vi "RT Loop - Data Logging.vi"(0 "Message Queues":T1 caption="消息队列", 3 "error in (no error)":errorcluster caption="错误输入（无错误）") -> (10 "error out":errorcluster caption="错误输出")   [LabVIEW 2015]
uses:
  Support VIs/Message Queue/All Real-Time Message Queues.ctl
  Support VIs/Message Queue/Message Cluster.ctl
  Globals/Global - All RT Loop Stop.vi
  Globals/Global - Monitoring Variables.vi
  Globals/Global - RT Stream Connections.vi
  Globals/Global - Configuration Options.vi
  Support VIs/Message Queue/Message Queue.lvlib
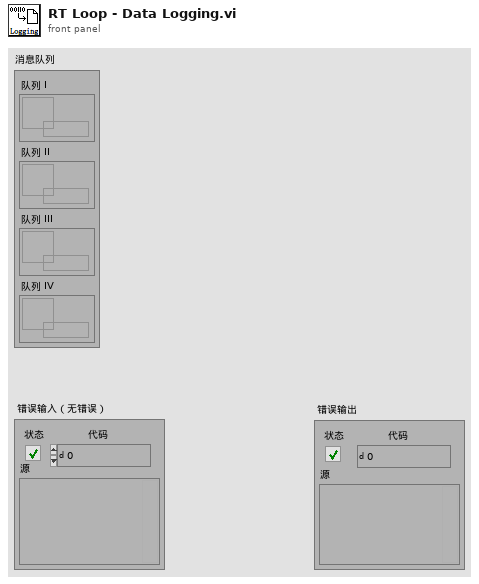
[diagram p1: front panel]
types:
  T1 = typedef "Message Queue.lvlib/All Real-Time Message Queues.ctl" = cluster{"Queue I":refnum<queue>, "Queue II":refnum<queue>, "Queue III":refnum<queue>, "Queue IV":refnum<queue>}
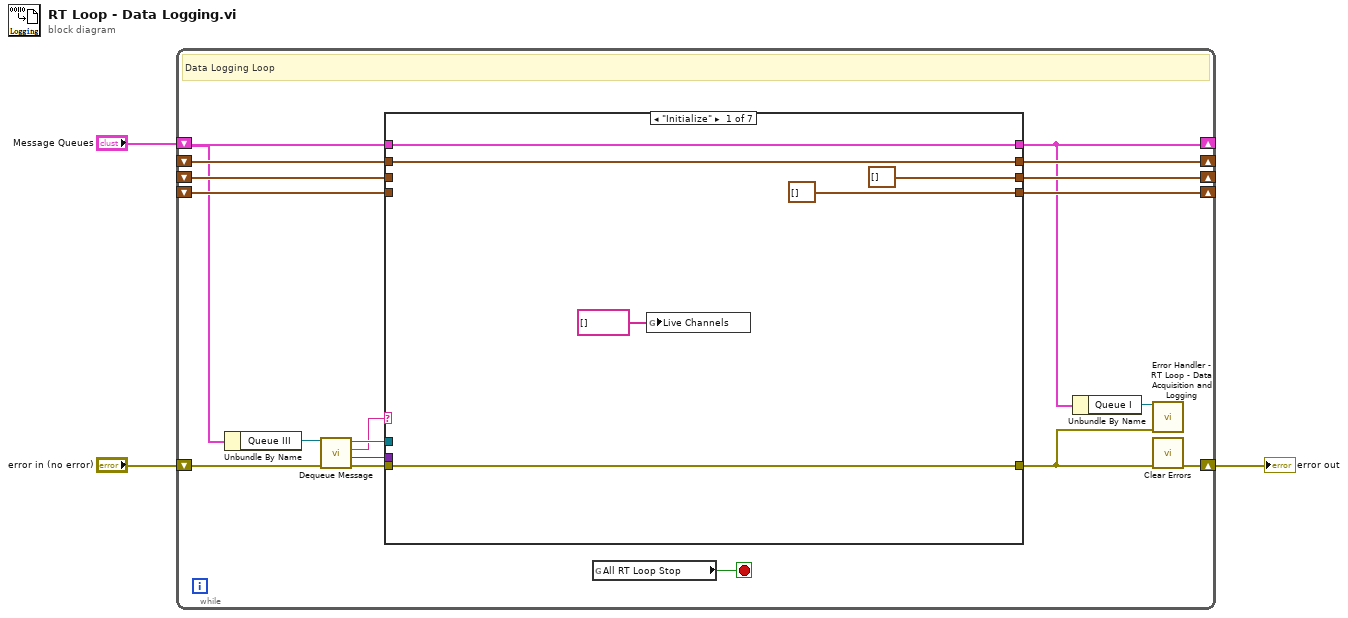
[diagram p0: block diagram]
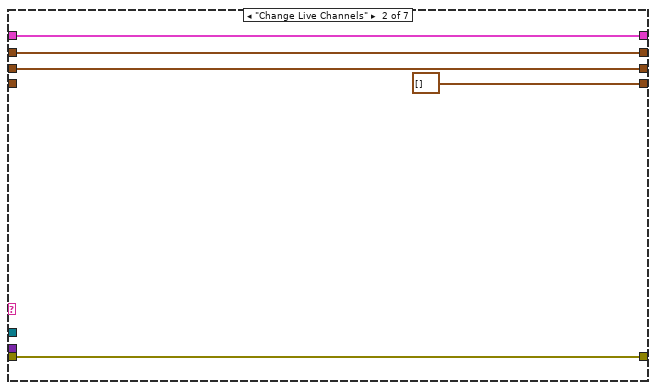
[diagram p2: hidden frame]
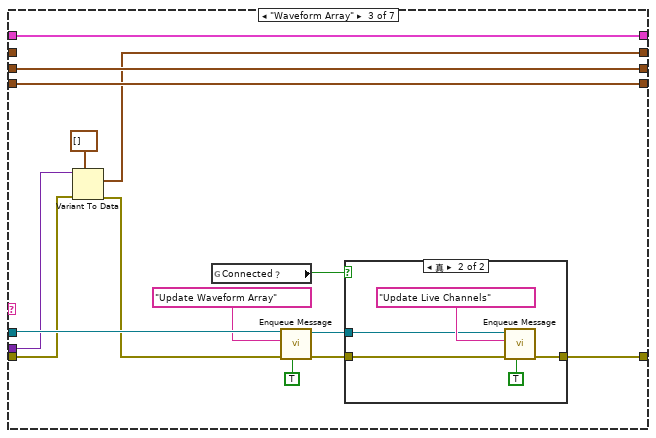
[diagram p3: hidden frame]
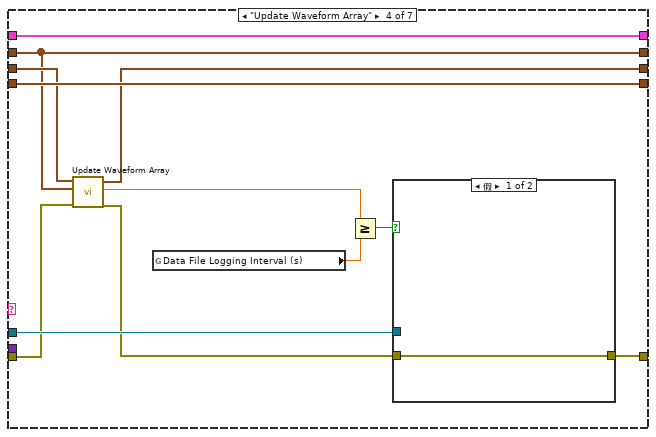
[diagram p5: hidden frame]
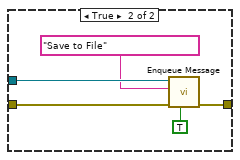
[diagram p6: hidden frame]
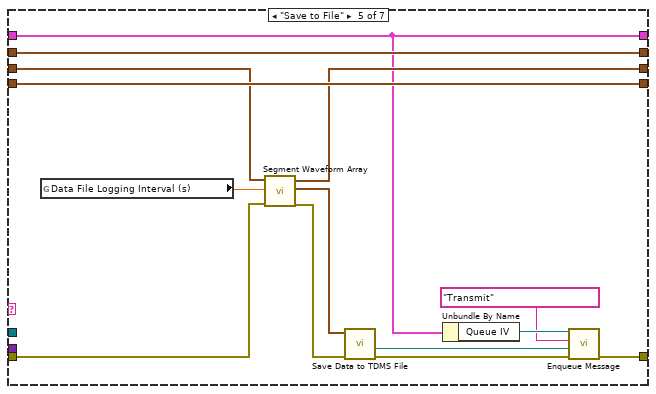
[diagram p7: hidden frame]
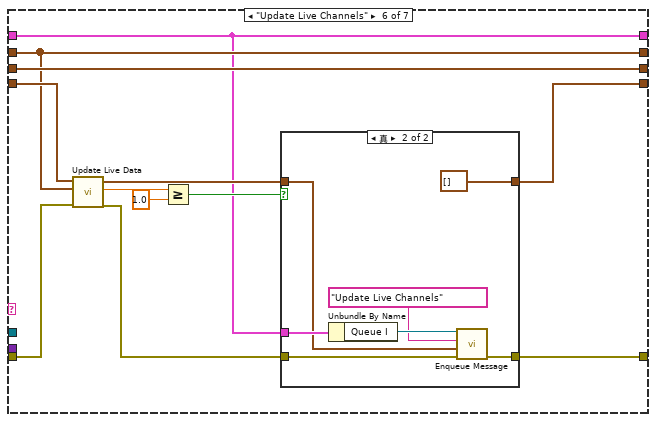
[diagram p8: hidden frame]
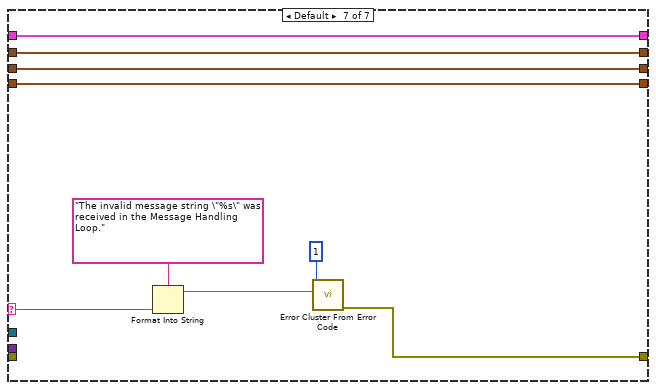
[diagram p10: hidden frame]
diagram:
  n1 = while {
    shift-right: [w17] -> _
    shift-left: _ -> [w10]
    shift-right: [w6] -> _
    shift-left: "Message Queues" -> [w7]
    shift-right: [w16] -> _
    shift-left: _ -> [w11]
    shift-right: [w12] -> w3
    shift-left: "error in (no error)" -> [w18]
    shift-right: [w8] -> _
    shift-left: _ -> [w9]
    stop <- w21 stop-if-true
    # "Data Logging Loop"
    n2 = Unbundle By Name(w7) -> ("Queue III"=w15:refnum<queue>)
    n3 = call "Dequeue Message.vi"("error in (no error)"=w18, "Message Queue"=w15) -> ("error out"=w20:errorcluster, "Message Data"=w19:variant, "Message"=w4:string, "dup Message Queue"=w5:refnum<queue>)  [unwired: 6 in]
    n4 = case shown="\"Initialize\"" w4 {
      tunnel: w19 -> [_ _ w45 _ _ _ _]
      selector: w4 -> [_ _ _ _ _ _ w112]
      tunnel: w20 -> [w24 w29 w46 w63 w77 w96 _]
      tunnel: [w26 w31 w33 w55 w80 w90 w109] -> w17
      tunnel: [w24 w29 w39 w58 w83 w97 w111] -> w13
      tunnel: w10 -> [w26 w31 _ w55 w80 w90 w109]
      tunnel: w7 -> [w27 w32 w35 w54 w72 w87 w110]
      tunnel: [w27 w32 w35 w54 w72 w87 w110] -> w6
      tunnel: [waveform(dbl)[] [] waveform(dbl)[] [] w43 w64 w85 w86 w108] -> w16
      tunnel: w11 -> [_ _ w43 w64 w85 w94 w108]
      tunnel: w9 -> [_ w30 w34 w62 w79 w91 w107]
      tunnel: [waveform(dbl)[] [] w30 w34 w61 w76 w91 w107] -> w8
      tunnel: w5 -> [_ _ w47 w65 _ _ _]
      frame "Initialize" {
        n5 = global write "Global - Monitoring Variables.vi" "Live Channels"(string[] [] ("Live Channels")) -> ()
      }
      frame "Change Live Channels" {
      }
      frame "Waveform Array" {
        n6 = Variant To Data(error in=w46, type=waveform(dbl)[] [], Variant=w45) -> (data=w33:waveform(dbl)[], error out=w36:errorcluster)
        n7 = global read "Global - RT Stream Connections.vi" "Connected？"() -> (w42:bool)
        n8 = call "Enqueue Message.vi"("Priority Message? (F)"=TRUE, "error in (no error)"=w36, "Message"="Update Waveform Array", "Message Queue"=w47) -> ("error out"=w41:errorcluster, "dup Message Queue"=w40:refnum<queue>)  [unwired: 6 in]
        n9 = case shown="真" w42 {
          tunnel: w41 -> [w48 w53]
          tunnel: [w48 w52] -> w39
          tunnel: w40 -> [_ w49]
          frame False {
          }
          frame True {
            n10 = call "Enqueue Message.vi"("Priority Message? (F)"=TRUE, "error in (no error)"=w53, "Message"="Update Live Channels", "Message Queue"=w49) -> ("error out"=w52:errorcluster)  [unwired: 6 in, 1 out]
          }
        }
      }
      frame "Update Waveform Array" {
        n11 = call "Update Waveform Array.vi"("error in (no error)"=w63, "new waveform array"=w55, "original waveform array"=w62) -> ("error out"=w57:errorcluster, "min duration"=w60:dbl, "updated wavefrom array"=w61:waveform(dbl)[])  [unwired: 6 in]
        n12 = global read "Global - Configuration Options.vi" "Data File Logging Interval (s)"() -> (w59:dbl)
        n13 = Greater Or Equal?(x=w60, y=w59) -> (x >= y?=w56:bool)
        n14 = case shown="假" w56 {
          tunnel: [w66 w70] -> w58
          tunnel: w57 -> [w66 w71]
          tunnel: w65 -> [_ w68]
          frame False {
          }
          frame True {
            n15 = call "Enqueue Message.vi"("Priority Message? (F)"=TRUE, "error in (no error)"=w71, "Message"="Save to File", "Message Queue"=w68) -> ("error out"=w70:errorcluster)  [unwired: 6 in, 1 out]
          }
        }
      }
      frame "Save to File" {
        n16 = global read "Global - Configuration Options.vi" "Data File Logging Interval (s)"() -> (w75:dbl)
        n17 = call "Segment Waveform Array.vi"("error in (no error)"=w77, "segment time"=w75, "original wavefrom array"=w79) -> ("error out"=w78:errorcluster, "waveform array part 0"=w73:waveform(dbl)[], "waveform array part 1"=w76:waveform(dbl)[])  [unwired: 6 in]
        n18 = call "Save Data to TDMS File.vi"("error in (no error)"=w78, "Waveform Data Array"=w73) -> ("error out"=w84:errorcluster, "Completed file path"=w74:path)  [unwired: 8 in]
        n19 = Unbundle By Name(w72) -> ("Queue IV"=w82:refnum<queue>)
        n20 = call "Enqueue Message.vi"("error in (no error)"=w84, "Message Data"=w74, "Message"="Transmit", "Message Queue"=w82) -> ("error out"=w83:errorcluster)  [unwired: 6 in, 1 out]
      }
      frame "Update Live Channels" {
        n21 = call "Update Live Data.vi"("error in (no error)"=w96, "new waveform array"=w90, "original waveform array"=w94) -> ("error out"=w95:errorcluster, "min duration"=w89:dbl, "updated wavefrom array"=w92:waveform(dbl)[])  [unwired: 6 in]
        n22 = Greater Or Equal?(x=w89, y=1.0) -> (x >= y?=w93:bool)
        n23 = case shown="真" w93 {
          tunnel: w95 -> [w99 w106]
          tunnel: [w99 w105] -> w97
          tunnel: w87 -> [_ w104]
          tunnel: w92 -> [w98 w101]
          tunnel: [w98 waveform(dbl)[] []] -> w86
          frame False {
          }
          frame True {
            n24 = Unbundle By Name(w104) -> ("Queue I"=w103:refnum<queue>)
            n25 = call "Enqueue Message.vi"("error in (no error)"=w106, "Message Data"=w101, "Message"="Update Live Channels", "Message Queue"=w103) -> ("error out"=w105:errorcluster)  [unwired: 6 in, 1 out]
          }
        }
      }
      frame Default {
        n26 = Format Into String(format string="The invalid message string \"%s\" was received in the Message Handling Loop." ("Unknown Message Error Text"), w112) -> (resulting string=w113:string)  [unwired: 2 in, 1 out]
        n27 = call <vilib>:"Error Cluster From Error Code.vi"("error message (\"\")"=w113, "error code (0)"=1) -> ("error out"=w111:errorcluster)  [unwired: 7 in]
      }
    }
    n28 = global read "Global - All RT Loop Stop.vi" "All RT Loop Stop"() -> (w21:bool)
    n29 = Unbundle By Name(w6) -> ("Queue I"=w14:refnum<queue>)
    n30 = call "Error Handler - RT Loop - Data Acquisition and Logging.vi"("error in (no error)"=w13, "Message Queue"=w14) -> ()  [unwired: 9 in, 1 out]
    n31 = call <vilib>:"Clear Errors.vi"("error in (no error)"=w13) -> ("error out"=w12:errorcluster)  [unwired: 5 in, 1 out]
  }
  "error out" <- w3
